vi "FGCTYdll.vi"(8 "error in (no error)":errorcluster, 9 "z":dbl[](array[numeric]), 10 "D":dbl, 11 "t":dbl) -> (0 "error out":errorcluster, 3 "f out":dbl[](array[numeric]))   [LabVIEW 2015]
doc: "subroutine FGCTY (t,D,z,f)\n\nOld routine to compute fugacity for each of the nc components of a mixture\nby numerical differentiation (using central differences) of the\ndimensionless residual Helmholtz energy.\n\nbased on derivations in E.W. Lemmon, MS Thesis, University of Idaho\n(1991); section 3.2\n\nINPUTS:\n t--temperature [K]\n D--molar density [mol/L]\n z--composition [array of mol frac]\n\nOUTPUTS:\n f--array (1..nc) of fugacities [kPa]"
uses:
  REFPROP.dll
panel:
  # "REFPROP-FGCTYdll.vi"
  # "void  FGCTYdll(double *t, double *D, double *z, double *f)"
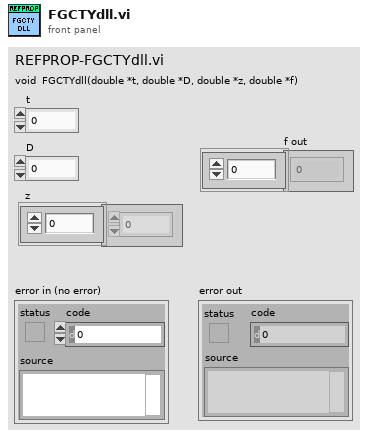
[diagram p1: front panel]
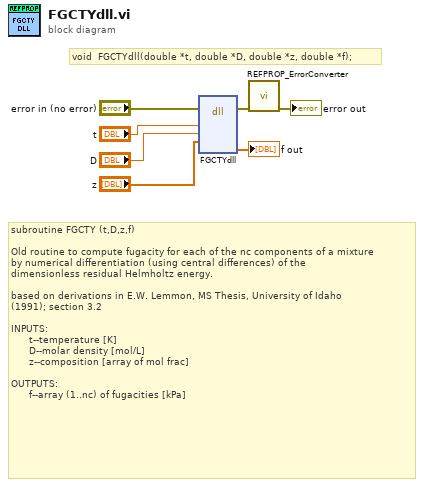
[diagram p0: block diagram]
diagram:
  # "void  FGCTYdll(double *t, double *D, double *z, double *f);"
  # "subroutine FGCTY (t,D,z,f)\n\nOld routine to compute fugacity for each of the nc components of a mixture\nby numerical differentiation (using central differences) of the\ndimensionless residual Helmholtz energy.\n\nbased on derivations in E.W. Lemmon, MS Thesis, University of Idaho\n(1991); section 3.2\n\nINPUTS:\n      t--temperature [K]\n      D--molar density [mol/L]\n      z--composition [array of mol frac]\n\nOUTPUTS:\n      f--array (1..nc) of fugacities [kPa]"
  n1 = dll-call lib="C:/Users/lauria/Desktop/REFPROP 10 LabVIEW Wrapper BETA/REFPROP/REFPROP.*" fn="FGCTYdll"(error in="error in (no error)", "t"="t", "D"="D", "z"="z") -> (error out=w3:errorcluster, "f"=→"f out":dbl[])  [unwired: 7 in, 1 out]
  n2 = call "REFPROP_ErrorConverter.vi"("error in (no error)"=w3) -> ("error out"=→"error out":errorcluster)  [unwired: 10 in]
